vi "Configure IF Bandwith.vi"(8 "error in (no error)":errorcluster, 10 "IF BW [Hz]":dbl, 11 "VNA-Ag87xx in":refnum<class "VNA-Ag87xx.lvclass">) -> (0 "error out":errorcluster, 2 "IF BW used [Hz]":dbl, 3 "VNA-Ag87xx out":refnum<class "VNA-Ag87xx.lvclass">)   [LabVIEW 2020, in "VNA-Ag87xx.lvclass"]
doc: "Configures the Intermidiate Frequency Bandwidth. \nIt chooses the closest supported bandwidth.\nIt returns the used IF BW."
uses:
  VNA-Ag87xx.lvclass
  C:/Sandbox/RF Bench/Source Code/WiSpry Test Framework/Instruments/Instrument.lvclass
  C:/Sandbox/RF Bench/Source Code/WiSpry Test Framework/Instruments/Vector Network Analyzer/Vector Network Analyzer.lvclass
  Instrument.lvclass/Instrument.ctl
  Vector Network Analyzer.lvclass/Vector Network Analyzer.ctl
  Instrument.lvclass
  Vector Network Analyzer.lvclass
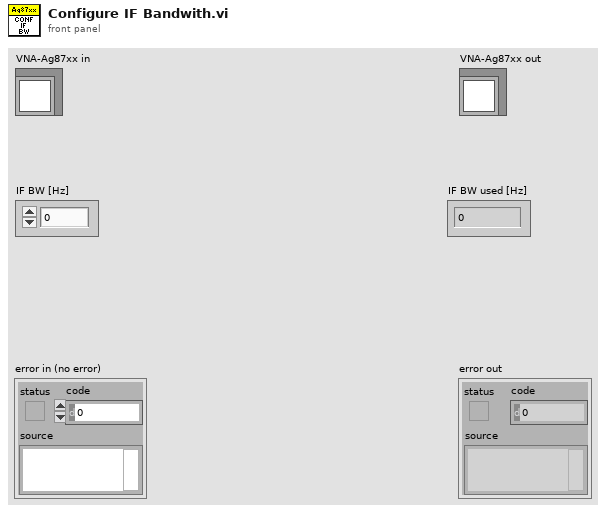
[diagram p1: front panel]
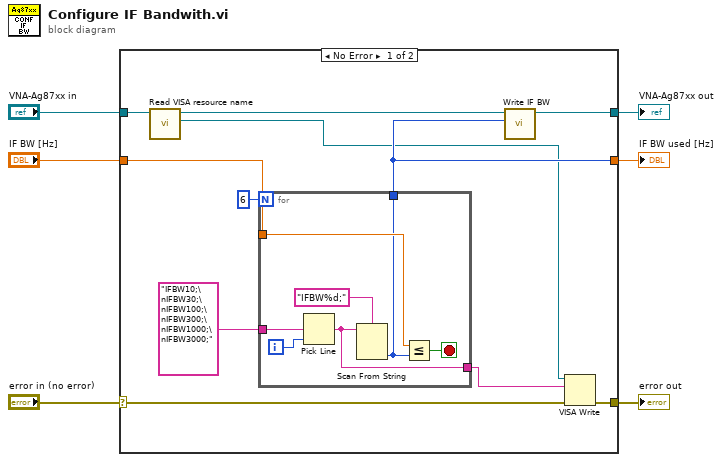
[diagram p0: block diagram]
diagram:
  n1 = case shown="No Error" "error in (no error)" {
    selector: "error in (no error)" -> [w13 w26]
    tunnel: [w15 w27] -> w5
    tunnel: "VNA-Ag87xx in" -> [w17 w27]
    tunnel: [w14 w26] -> w6
    tunnel: "IF BW [Hz]" -> [w11 w25]
    tunnel: [w10 w25] -> w1
    frame No Error {
      n2 = call "Read VISA resource name.vi"("Instrument in"=w17) -> ("VISA resource name"=w7:refnum<visa-resource-name>, "Instrument out"=w16:refnum<class "VNA-Ag87xx.lvclass">)  [unwired: 9 in]
      n3 = for {
        N: 6 -> [_]
        tunnel: "IFBW10;\nIFBW30;\nIFBW100;\nIFBW300;\nIFBW1000;\nIFBW3000;" -> [w24]
        tunnel: w11 -> [w21]
        tunnel: [w18] -> w8
        tunnel: [w19] -> w10
        i -> [w23]
        stop <- w20 stop-if-true
        n4 = Pick Line(multi-line string=w24, line index=w23) -> (output string=w18:string)  [unwired: 1 in]
        n5 = Scan From String(format string="IFBW%d;", input string=w18) -> (output 1=w19:i32)  [unwired: 3 in, 3 out]
        n6 = Less Or Equal?(x=w21, y=w19) -> (x <= y?=w20:bool)
      }
      n7 = call "Write IF BW.vi"("IF BW"=w10, "Vector Network Analyzer in"=w16) -> ("Vector Network Analyzer out"=w15:refnum<class "VNA-Ag87xx.lvclass">)  [unwired: 9 in]
      n8 = VISA Write(VISA resource name=w7, write buffer=w8, error in (no error)=w13) -> (error out=w14:errorcluster)  [unwired: 2 out]
    }
    frame Error {
    }
  }
  "error out" <- w6
  "VNA-Ag87xx out" <- w5
  "IF BW used [Hz]" <- w1
